vi "Measurement Logic.vi"() -> ()   [LabVIEW 2021, in "Load Transient Response with Pin Map.lvlib"]
uses:
  Load Transient Response with Pin Map.lvlib
  <vilib>/Plug-In SDKs/Measurements/Measure Call Context/Measure Call Context.lvclass
  Measurement Configuration.ctl
  <instrlib>/niScope/Controls/niScope vertical coupling.ctl
  Measurement Results.ctl
  subVIs/Reference values.ctl
  <vilib>/Plug-In SDKs/Clients/Session Management V1/Session Reservation/Session Reservation.lvclass
  common/Instrument Control/Scope/TClk/Instrument Info.ctl
  common/Instrument Control/Scope Parameters.ctl
  <instrlib>/niDCPower/nidcpower.llb/niDCPower Sense.ctl
  <instrlib>/niDCPower/nidcpower.llb/niDCPower Source Mode.ctl
  <instrlib>/niDCPower/nidcpower.llb/niDCPower Wait For Event - Event.ctl
  <instrlib>/niDCPower/nidcpower.llb/niDCPower Output Function.ctl
  <instrlib>/niDCPower/nidcpower.llb/niDCPower Aperture Time Units.ctl
  <vilib>/Plug-In SDKs/Measurements/Measure Call Context/Reserve Sessions - NPin.vi
  <vilib>/Plug-In SDKs/Sessions/niDCPower/Initialize Sessions - NSess.vi
  <vilib>/Plug-In SDKs/Sessions/niDCPower/Get Connections - 1Pin 1Conn.vi
  <vilib>/Plug-In SDKs/Sessions/niScope/Initialize Sessions - NSess.vi
  <vilib>/Plug-In SDKs/Sessions/niScope/Get Connections - NPin MConn.vi
  <instrlib>/niScope/Configure/Trigger/niScope Configure Trigger Digital.vi
  <instrlib>/niDCPower/nidcpower.llb/niDCPower Configure Digital Edge Measure Trigger With Channels.vi
  <vilib>/Plug-In SDKs/Sessions/niDCPower/NI Session Management niDCPower.lvlib
  <vilib>/Plug-In SDKs/Sessions/niScope/NI Session Management niScope.lvlib
  common/PMIC Common.lvlib
panel:
  out "measurement results":T1={"Status"="Empty", "dt"=0.0, "Load voltages"=[0.0], "Load currents"=[0.0], "Undershoot load voltage"=0.0, "Overshoot load voltage"=0.0, "waveform pins"=[], "waveform sites"=[], "waveform t0 array"=[], "waveform dt array"=[], "waveform length array"=[], "concatenated waveform Y"=[]}
  in  "measurement configuration":T2={"Mode of operation"=enum."Perform measurement", "DUT setup time"=1.2, "Nominal output voltage"=32.0, "Source pin name"="Lorem ipsum dolor sit", "Source sense"=64, "Source current limit"=64.0, "Source voltage level"=-32.0, "Source transient response"=-32, "Source voltage gain bandwidth"=-64.0, "Source voltage compensation frequency"=-64.0, "Source voltage pole-zero ratio"=1.0, "Load pin name"="Lorem ipsum dolor sit", "Load sense"=1, "Load voltage limit range"=1.0, "Load current level range"=40.0, "Load sample rate"=1800000.0, "Load current set point 1"=4.0, "Load current set point 2"=14.0, "Load current delay t1"=0.001, "Load current pulse duration"=0.001, "Load current delay t2"=0.001, "Load current rising slew rate"=24.0, "Load current falling slew rate"=24.0, "Load transient response"=1042, "Load current gain bandwidth"=14000.0, "Load current compensation frequency"=180000.0, "Load current pole-zero ratio"=0.3, "Pin Names for Scope"=[], "vertical range"=[], "vertical offset"=[], "probe attenuation"=[], "vertical coupling"=[], "input impedance"=[], "max input frequency"=[], "min record length"=[], "channel enabled"=[], "enforce realtime"=[], "reference position"=[], "min sample rate"=[]} {"input impedance" items=["1 mega ohm"=0, "50 ohms"=2]; "vertical coupling" items=["AC", "DC", "Ground"]; "Load transient response" items=["Slow"=1041, "Normal"=1038, "Fast"=1039, "Custom"=1042]; "Load current falling slew rate" format="%#_6p"; "Load current rising slew rate" format="%#_6p"; "Load current level range" format="%#_6p"; "Load voltage limit range" format="%#_6p"; "Load sense" items=["Red", "Green", "Blue"]; "Source transient response" items=["Slow"=1041, "Normal"=1038, "Fast"=1039, "Custom"=1042]; "Source sense" items=["Local"=1008, "Remote"=1009]; "Nominal output voltage" format="%#_6pV"}
  out "measure call context out":refnum<class "Measure Call Context.lvclass">
  in  "measure call context in":refnum<class "Measure Call Context.lvclass">
  out "error out":errorcluster
  in  "error in":errorcluster
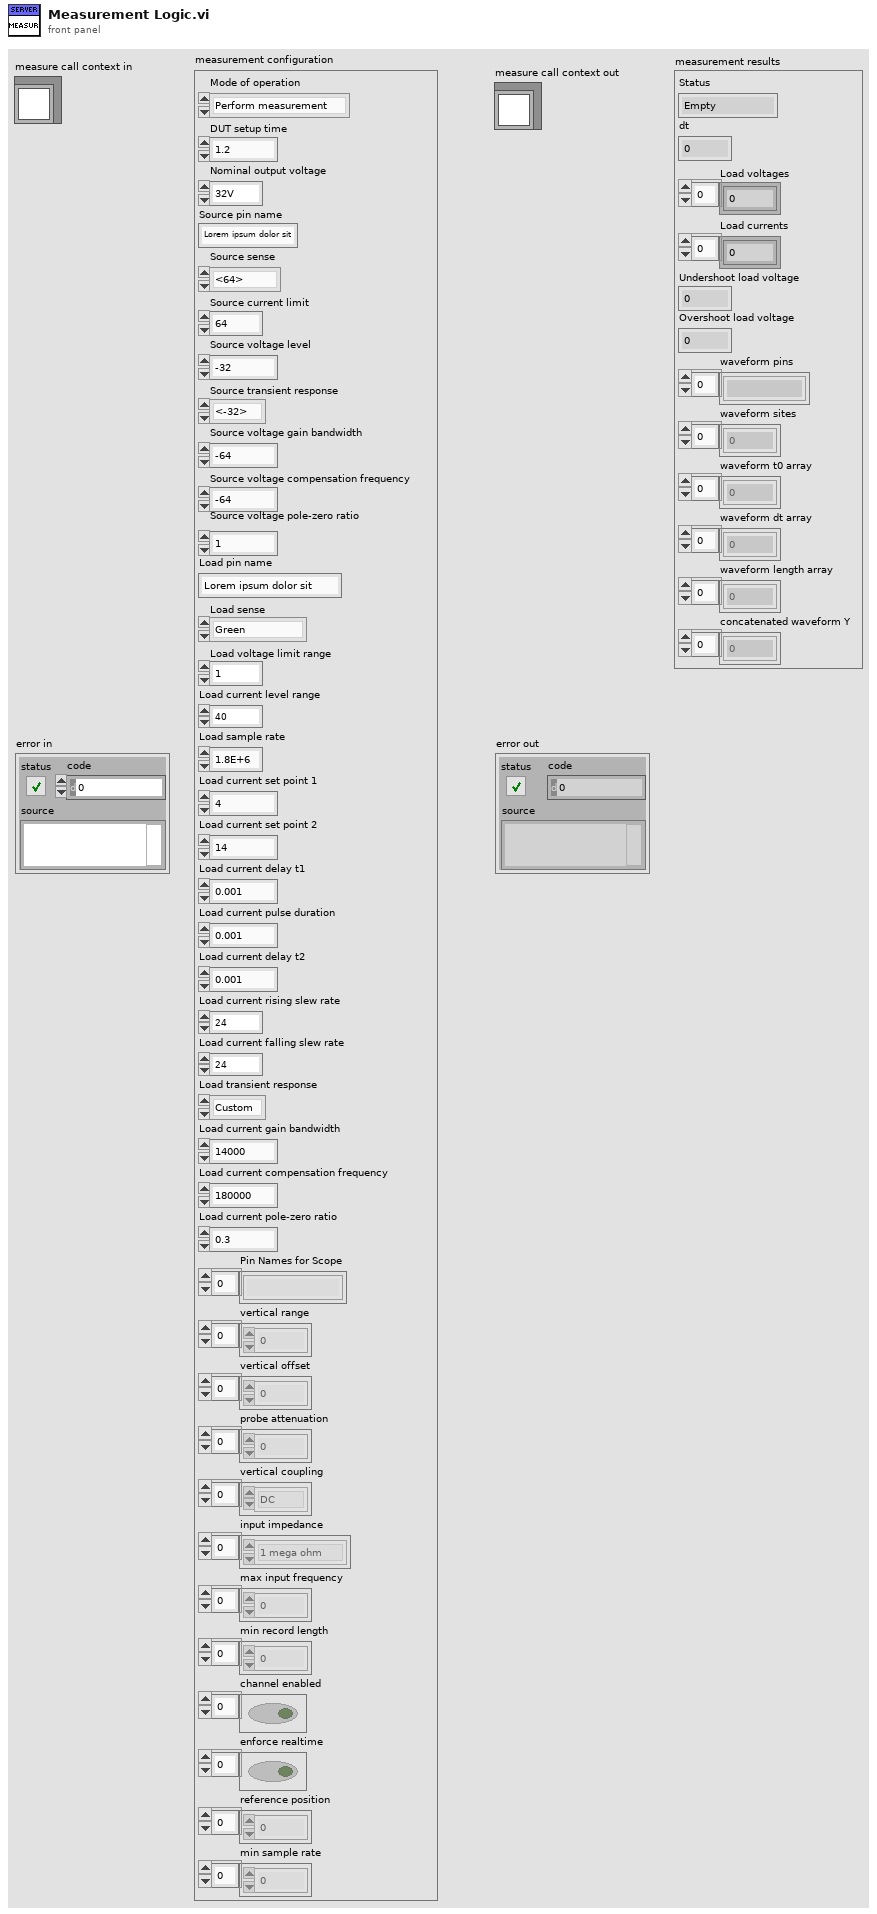
[diagram p1: front panel]
types:
  T1 = typedef "Load Transient Response with Pin Map.lvlib/Measurement Results.ctl" = cluster{"Status":string, "dt":dbl, "Load voltages":dbl[], "Load currents":dbl[], "Undershoot load voltage":dbl, "Overshoot load voltage":dbl, "waveform pins":string[], "waveform sites":i32[], "waveform t0 array":dbl[], "waveform dt array":dbl[], "waveform length array":i32[], "concatenated waveform Y":dbl[]}
  T2 = typedef "Load Transient Response with Pin Map.lvlib/Measurement Configuration.ctl" = cluster{"Mode of operation":enum32{"Power on the DUT", "Perform measurement", "Power off the DUT"}, "DUT setup time":dbl, "Nominal output voltage":dbl, "Source pin name":string, "Source sense":i32, "Source current limit":dbl, "Source voltage level":dbl, "Source transient response":i32, "Source voltage gain bandwidth":dbl, "Source voltage compensation frequency":dbl, "Source voltage pole-zero ratio":dbl, "Load pin name":string, "Load sense":i32, "Load voltage limit range":dbl, "Load current level range":dbl, "Load sample rate":dbl, "Load current set point 1":dbl, "Load current set point 2":dbl, "Load current delay t1":dbl, "Load current pulse duration":dbl, "Load current delay t2":dbl, "Load current rising slew rate":dbl, "Load current falling slew rate":dbl, "Load transient response":i32, "Load current gain bandwidth":dbl, "Load current compensation frequency":dbl, "Load current pole-zero ratio":dbl, "Pin Names for Scope":string[], "vertical range":dbl[], "vertical offset":dbl[], "probe attenuation":dbl[], "vertical coupling":T3[], "input impedance":u32[], "max input frequency":dbl[], "min record length":i32[], "channel enabled":bool[], "enforce realtime":bool[], "reference position":dbl[], "min sample rate":dbl[]}
  T3 = typedef "niScope vertical coupling.ctl" = i32
  T4 = typedef "Load Transient Response with Pin Map.lvlib/Reference values.ctl" = cluster{"dcpower session reservation":refnum<class "Session Reservation.lvclass">, "Source out":refnum<k15>, "Source channel name":string, "Load out":refnum<k15>, "Load channel name":string, "No of samples to fetch":i32, "Source voltage level":dbl, "Source current limit":dbl, "Measure terminal name":string, "Scope ref trigger source":string, "scope session reservation":refnum<class "Session Reservation.lvclass">, "Scope handles":refnum<k15>[][], "connection map":map{string, T5[]}, "instrument info map array":map{string, cluster{"channel":string, "siteNumber":i32, "pin":string, "Scope Parameters":T6}[]}[], "Enable TClk":bool, "Number of records":i32, "Measurement Results":T1}
  T5 = typedef "PMIC Common.lvlib/Instrument Info.ctl" = cluster{"instrument":string, "channel":string, "siteNumber":i32}
  T6 = typedef "PMIC Common.lvlib/Scope Parameters.ctl" = cluster{"vertical range":dbl, "vertical offset":dbl, "probe attenuation":dbl, "vertical coupling":T3, "channel enabled":bool, "input impedance":u32, "maximum input frequency":dbl, "min sample rate":dbl, "reference position":dbl, "min record length":i32, "number of records":i32, "enforce realtime":bool}
  T7 = enum32{"Power on the DUT", "Perform measurement", "Power off the DUT"}
  T8 = typedef "niDCPower Wait For Event - Event.ctl" = i32
  T9 = typedef "niDCPower Source Mode.ctl" = i32
  T10 = typedef "niDCPower Sense.ctl" = i32
  T11 = typedef "NI Session Management niDCPower.lvlib/Connection with Session.ctl" = cluster{"connection":T12, "session":refnum<k15>}
  T12 = typedef "NI Session Management V1 Client.lvlib/Session Reservation.lvclass/Connection.ctl" = cluster{"pin or relay name":string, "site":i32, "instrument type id":string, "channel":string}
  T13 = typedef "niDCPower Output Function.ctl" = i32
  T14 = cluster{"Numeric":dbl, "Numeric":dbl, "Numeric":dbl, "vertical coupling":T3, "Boolean":bool, "input impedance":u32, "Numeric":dbl, "Numeric":dbl, "Numeric":dbl, "Numeric":i32, "Number of records":i32, "Boolean":bool}[]
  T15 = typedef "NI Session Management niScope.lvlib/Connection with Session.ctl" = cluster{"connection":T12, "session":refnum<k15>}
  T16 = typedef "NI Measurement Plug-In SDK.lvlib/Pin Map Context.ctl" = cluster{"pin map id":string, "sites":i32[]}
  T17 = map{string, cluster{"channel":string, "siteNumber":i32, "pin":string, "Scope Parameters":T6}[]}[]
  T18 = typedef "niDCPower Aperture Time Units.ctl" = i32
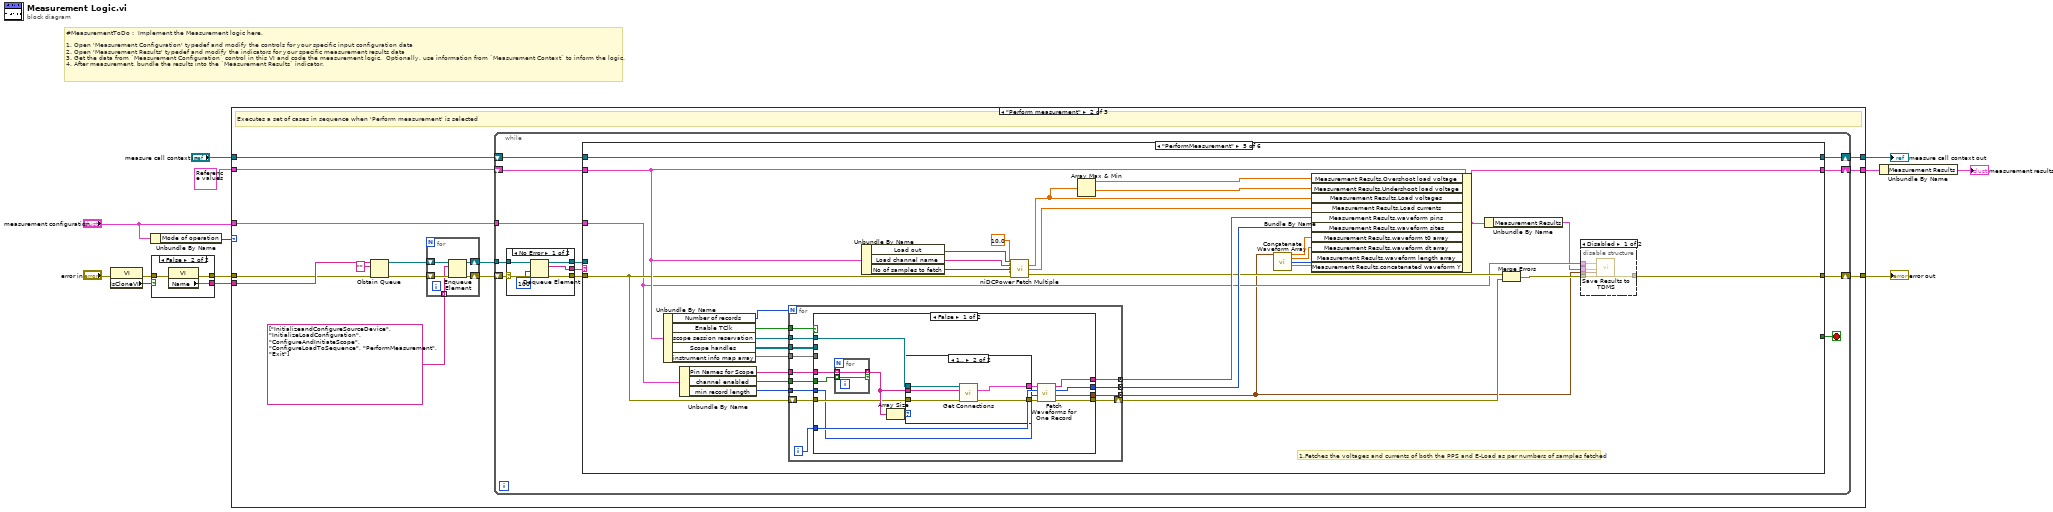
[diagram p0: block diagram]
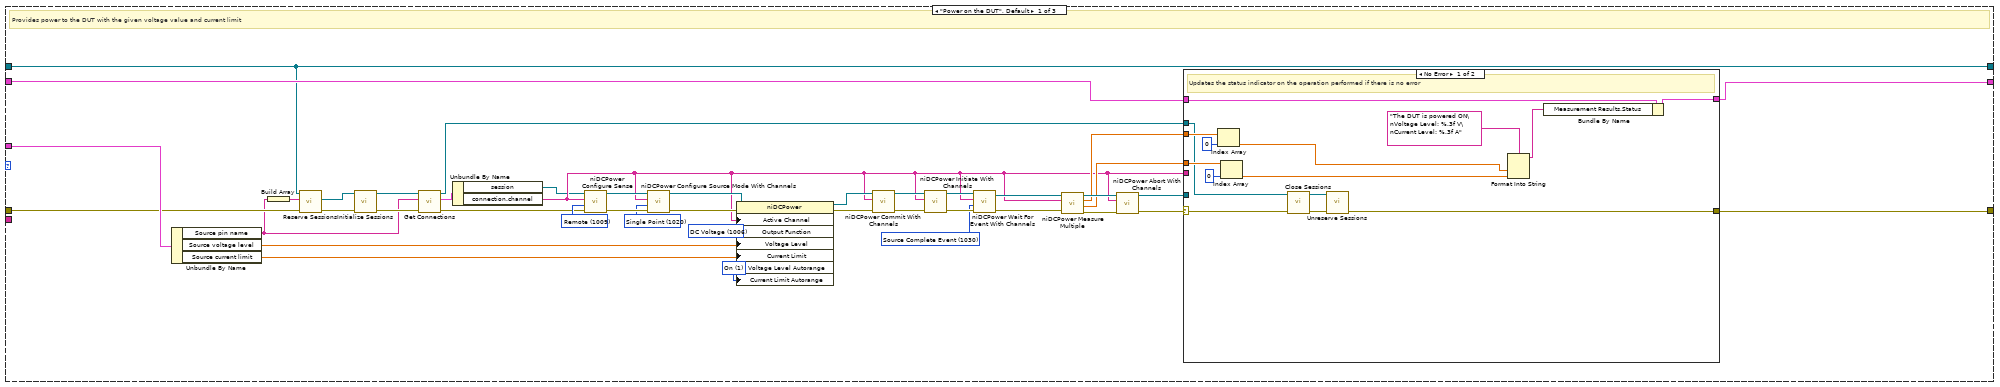
[diagram p2: hidden frame]
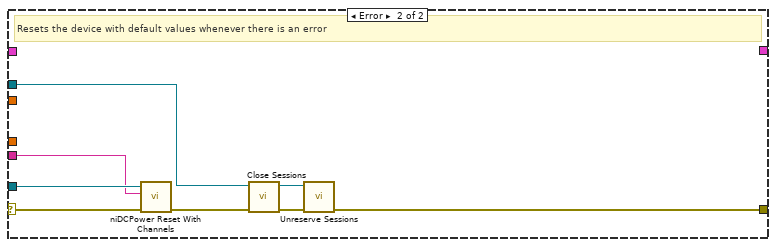
[diagram p3: hidden frame]
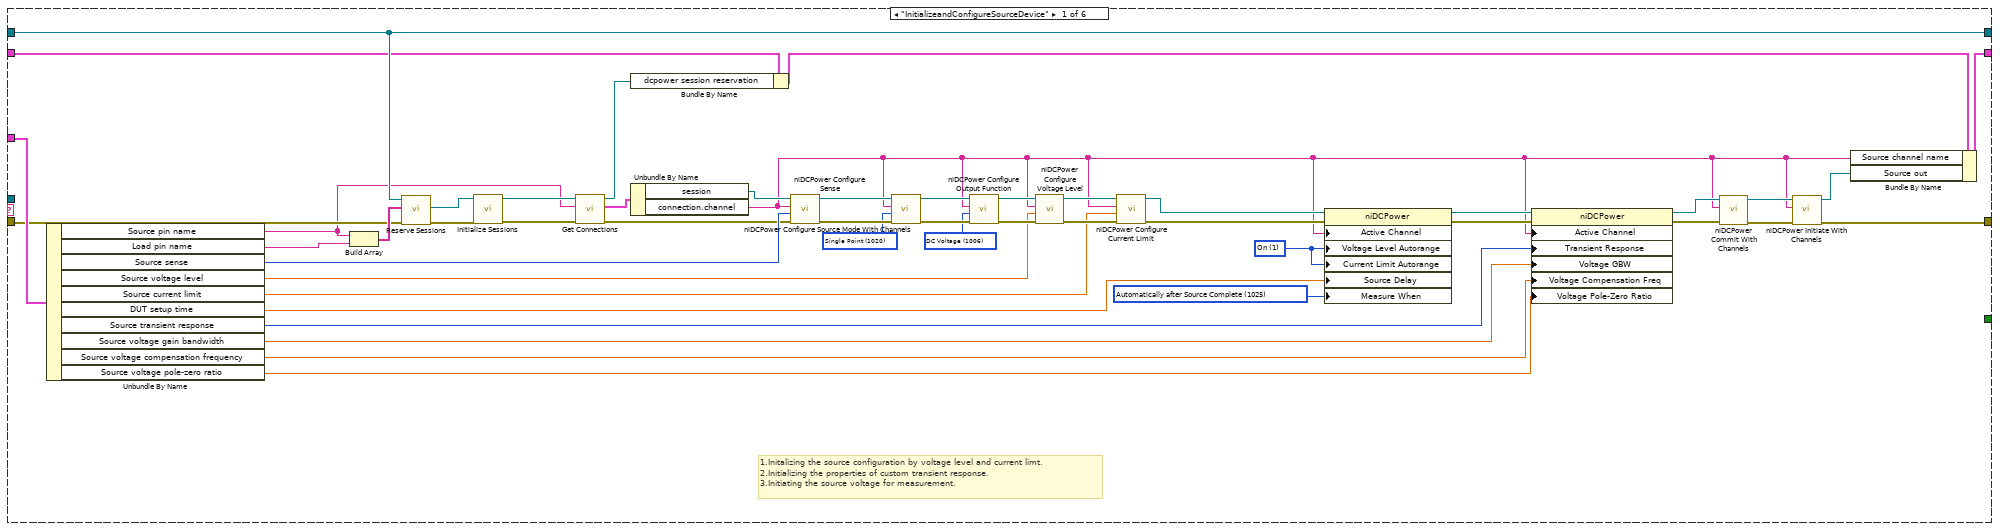
[diagram p4: hidden frame]
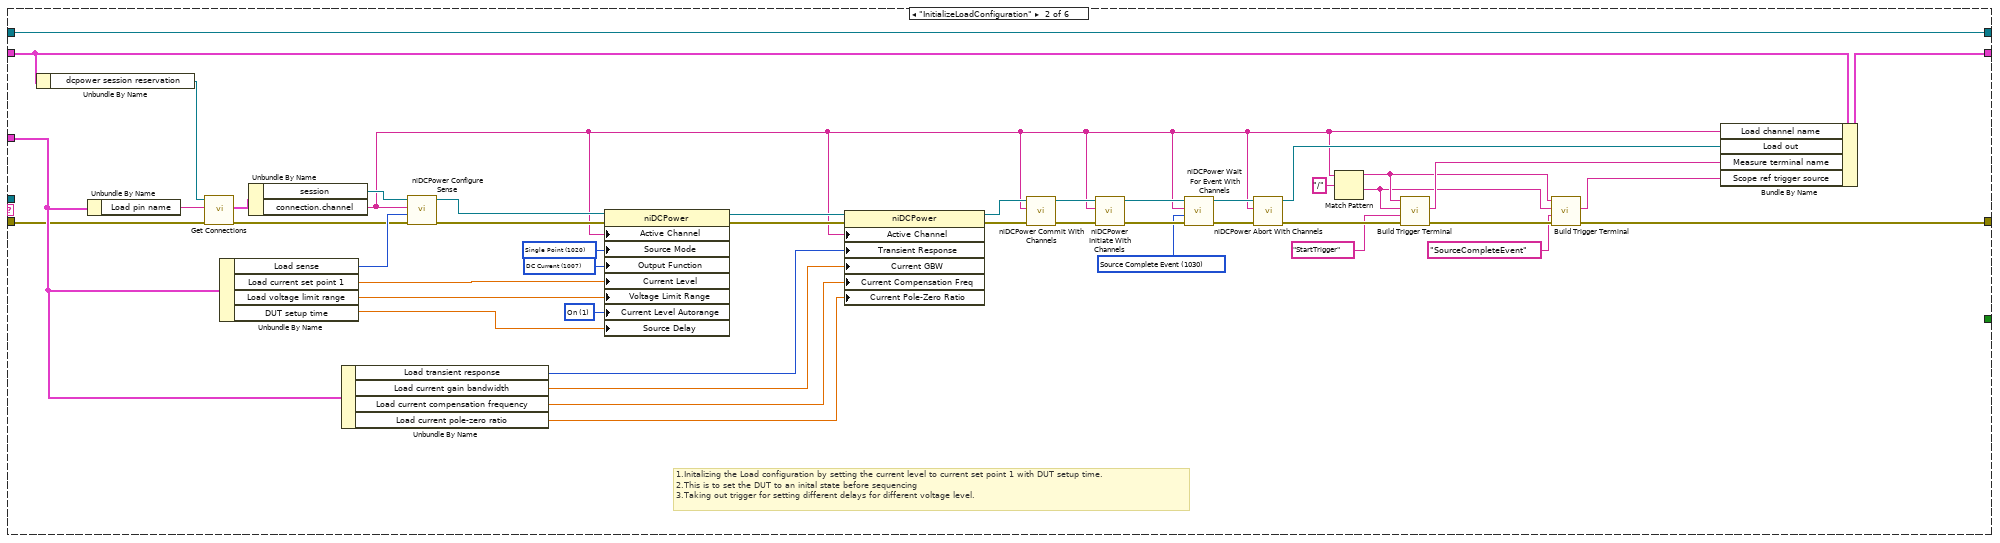
[diagram p5: hidden frame]
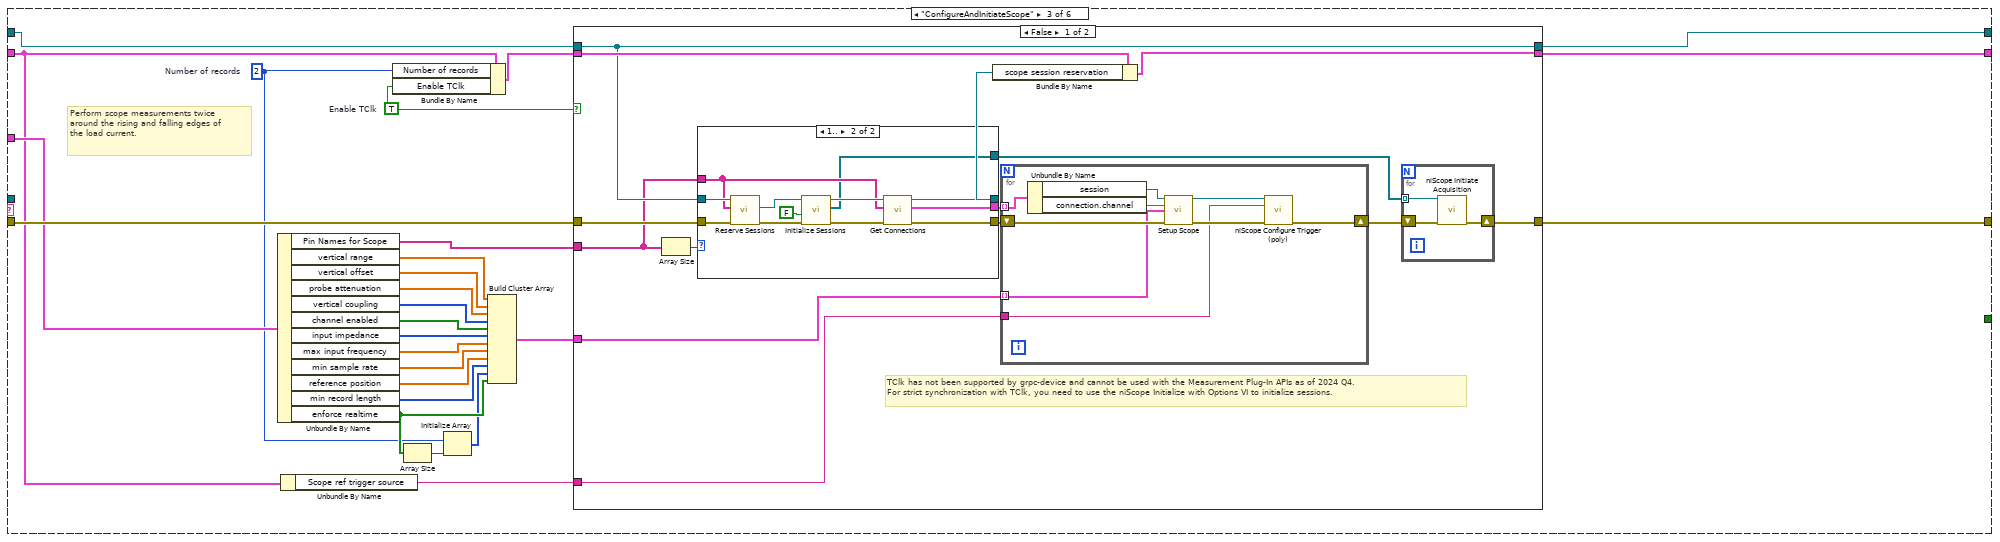
[diagram p6: hidden frame]
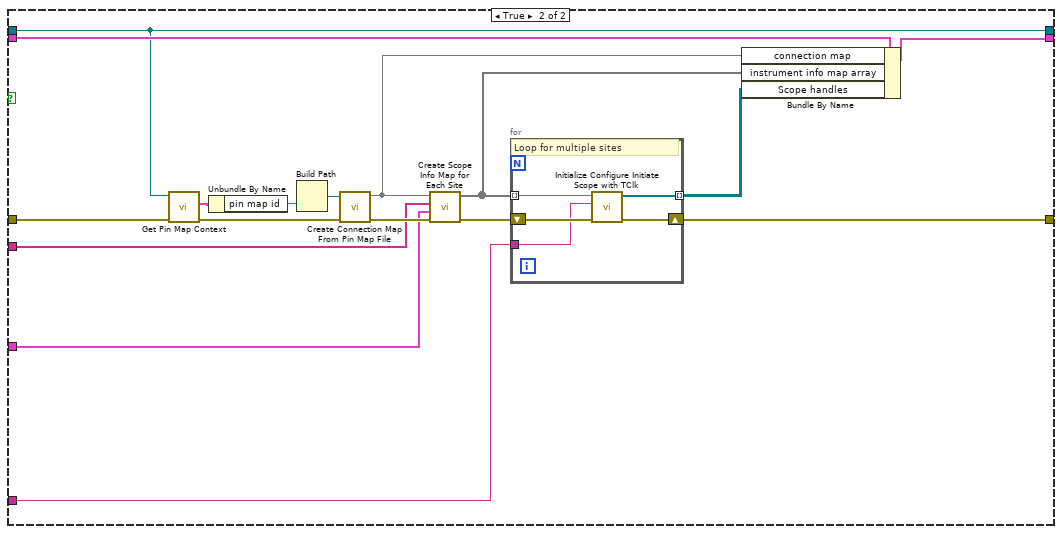
[diagram p8: hidden frame]
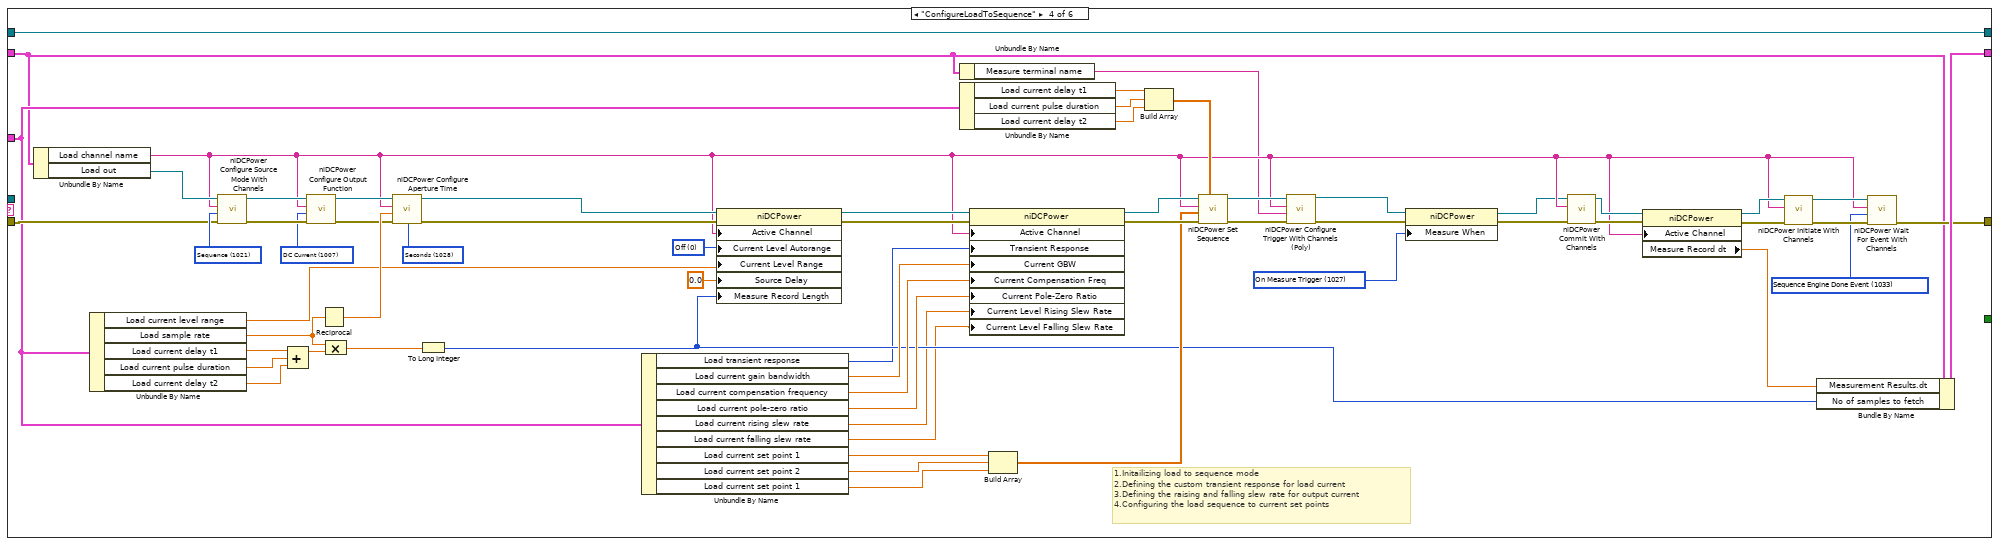
[diagram p9: hidden frame]
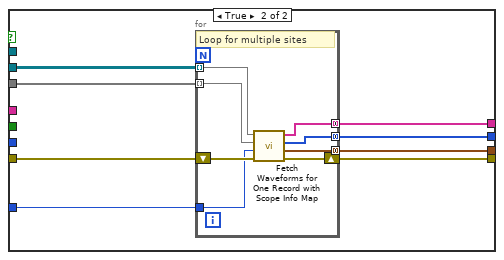
[diagram p12: hidden frame]
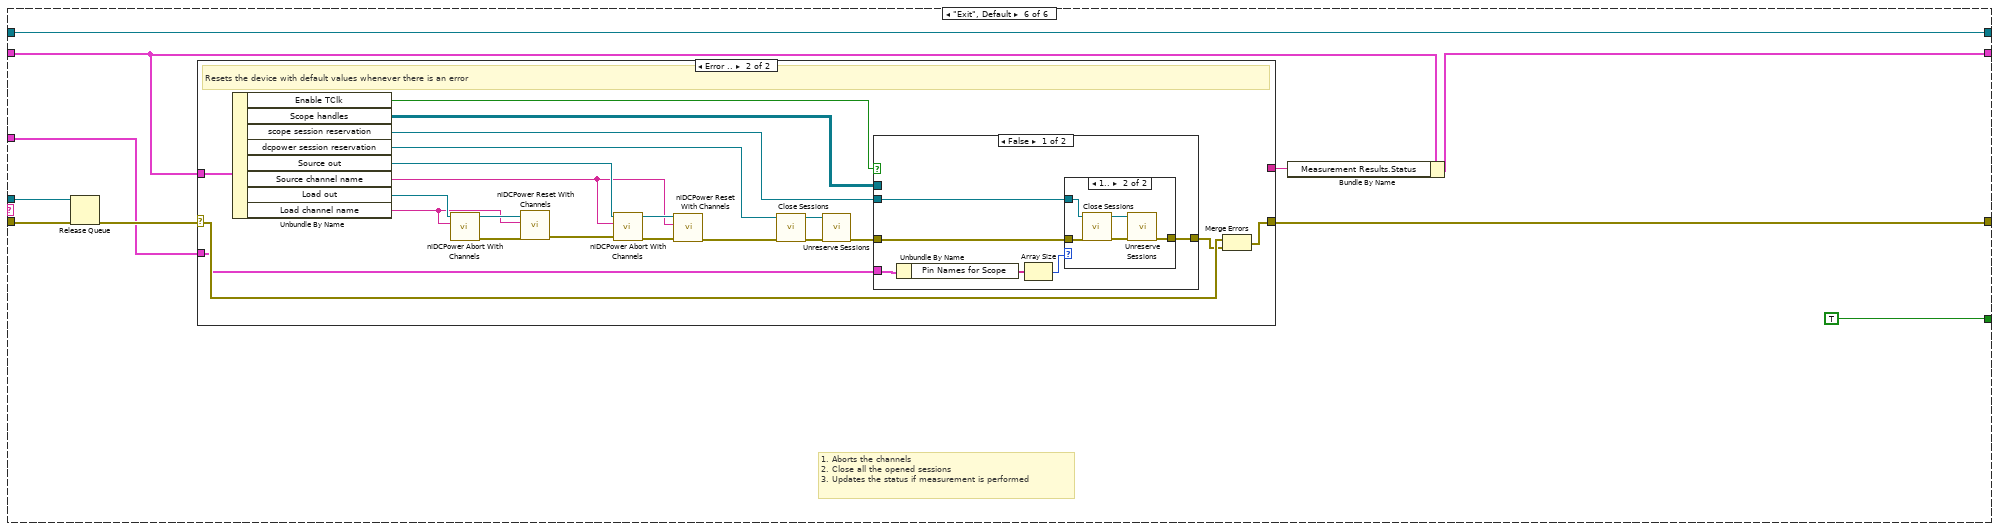
[diagram p13: hidden frame]
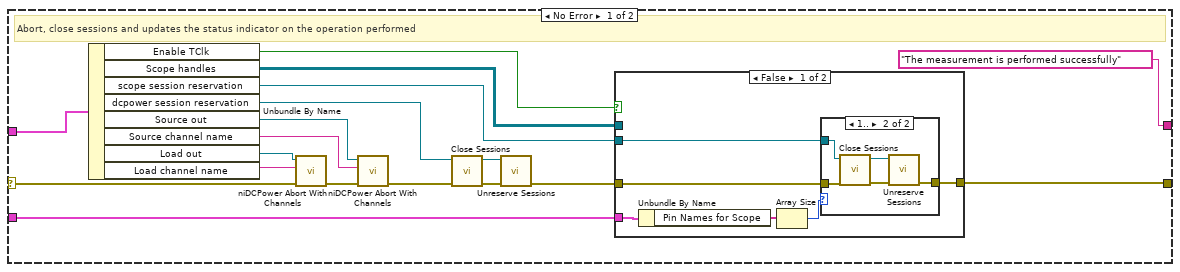
[diagram p14: hidden frame]
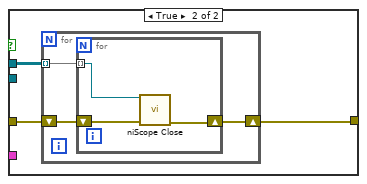
[diagram p16: hidden frame]
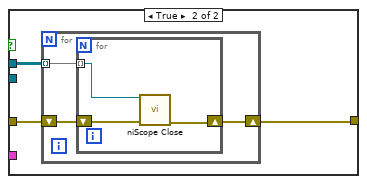
[diagram p18: hidden frame]
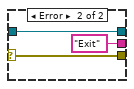
[diagram p19: hidden frame]
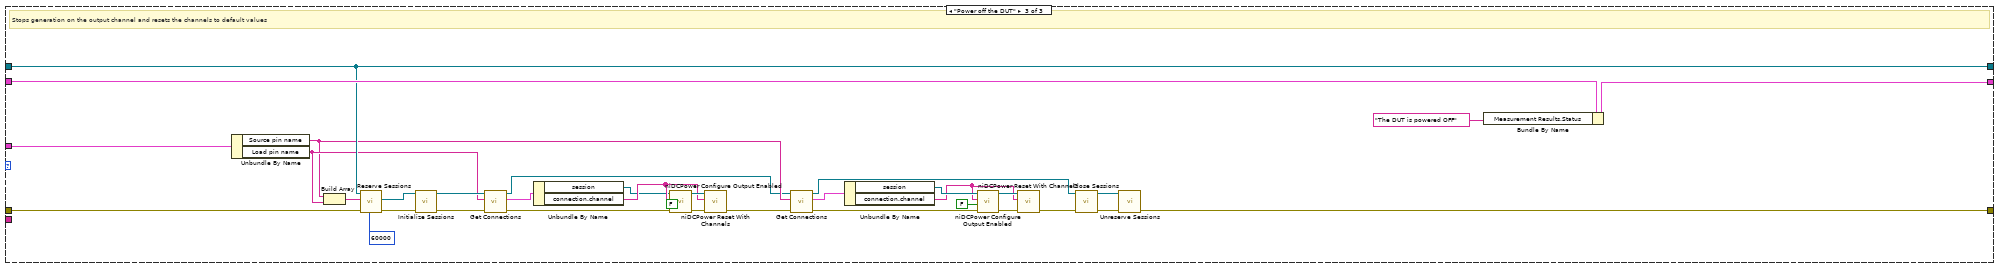
[diagram p20: hidden frame]
diagram:
  # "#MeasurementToDo :  Implement the Measurement logic here.\n\n1. Open 'Measurement Configuration' typedef and modify the controls for your specific input configuration data\n2. Open 'Measurement Results' typedef and modify the indicators for your specific measurement results data\n3. Get the data from `Measurement Configuration` control in this VI and code the measurement logic.  Optionally, use information from `Measurement Context` to inform the logic.\n4. After measurement, bundle the results into the `Measurement Results` indicator."
  n1 = property class="VI"(error in="error in") -> (error out=w12:errorcluster, "IsCloneVI"=w13:bool)  [unwired: 1 in, 1 out]
  n2 = Unbundle By Name("measurement configuration") -> ("Mode of operation"=w8:T7)
  n3 = case shown="False" w13 {
    tunnel: [w16 w19] -> w9
    tunnel: [w15 w18] -> w7
    tunnel: w12 -> [w14 w17]
    frame True {
      n4 = property class="VI"(error in=w14) -> (error out=w16:errorcluster, "Clone Name"=w15:string)  [unwired: 1 in, 1 out]
    }
    frame False {
      n5 = property class="VI"(error in=w17) -> (error out=w19:errorcluster, "Name"=w18:string)  [unwired: 1 in, 1 out]
    }
  }
  n6 = case shown="\"Perform measurement\"" w8 {
    tunnel: T4 {"dcpower session reservation"=refnum, "Source out"="", "Source channel name"="", "Load out"="", "Load channel name"="", "No of samples to fetch"=1, "Source voltage level"=0.0, "Source current limit"=0.0, "Measure terminal name"="", "Scope ref trigger source"="", "scope session reservation"=refnum, "Scope handles"=[], "connection map"={}, "instrument info map array"=[], "Enable TClk"=FALSE, "Number of records"=2, "Measurement Results"={"Status"="Empty", "dt"=0.0, "Load voltages"=[], "Load currents"=[], "Undershoot load voltage"=0.0, "Overshoot load voltage"=0.0, "waveform pins"=[], "waveform sites"=[], "waveform t0 array"=[], "waveform dt array"=[], "waveform length array"=[], "concatenated waveform Y"=[]}} -> [w41 w98 w580]
    tunnel: "measure call context in" -> [w28 w97 w570]
    tunnel: [w34 w96 w558] -> w1
    tunnel: [w28 w95 w570] -> w2
    tunnel: [w33 w94 w578] -> w10
    tunnel: "measurement configuration" -> [w44 w93 w581]
    tunnel: w9 -> [w26 w86 w572]
    tunnel: w7 -> [_ w89 _]
    frame "Power on the DUT", Default {
      w47 = 1 items=["Off", "On"] ("Source:DC Voltage:Voltage Level Autorange")
      w46 = T8 1030 items=["Source Complete Event"=1030, "Measure Complete Event"=1031, "Sequence Iteration Complete Event"=1032, "Sequence Engine Done Event"=1033, "Pulse Complete Event"=1051, "Ready For Pulse Trigger Event"=1052] ("event")
      w45 = T9 1020 items=["Single Point"=1020, "Sequence"=1021] ("source mode")
      w48 = 1006 items=["DC Voltage"=1006, "DC Current"=1007, "Pulse Voltage"=1049, "Pulse Current"=1050] ("Source:Output Function")
      w49 = T10 1009 items=["Local"=1008, "Remote"=1009] ("sense")
      # "Provides power to the DUT with the given voltage value and current limit"
      n7 = Unbundle By Name(w44) -> ("Source pin name"=w24:string, "Source voltage level"=w60:dbl, "Source current limit"=w61:dbl)
      n8 = Build Array(w24) -> (w27:string[])
      n9 = call-poly <vilib>:"Reserve Sessions.vi"("error in"=w26, "pin or relay names"=w27, "measurement context in"=w28) -> ("error out"=w32:errorcluster, "session reservation out"=w31:refnum<class "Session Reservation.lvclass">)  [unwired: 6 in, 1 out]
      n10 = call-poly <vilib>:"Initialize Sessions.vi"("error in"=w32, "session reservation in"=w31) -> ("error out"=w30:errorcluster, "session reservation out"=w29:refnum<class "Session Reservation.lvclass">)  [unwired: 6 in, 2 out]
      n11 = call-poly <vilib>:"Get Connections.vi"("error in"=w30, "pin or relay name"=w24, "session reservation in"=w29) -> ("error out"=w23:errorcluster, "connection"=w25:T11, "session reservation out"=w20:refnum<class "Session Reservation.lvclass">)  [unwired: 6 in]
      n12 = Unbundle By Name(w25) -> ("session"=w21:refnum<k15>, "connection.channel"=w22:string)
      n13 = call <instrlib>:"niDCPower Configure Sense.vi"("error in (no error)"=w23, "sense"=w49, "channel name"=w22, "instrument handle"=w21) -> ("error out"=w55:errorcluster, "instrument handle out"=w57:refnum<k15>)  [unwired: 6 in]
      n14 = call <instrlib>:"niDCPower Configure Source Mode With Channels.vi"("error in (no error)"=w55, "source mode"=w45, "channel name"=w22, "instrument handle"=w57) -> ("error out"=w54:errorcluster, "instrument handle out"=w56:refnum<k15>)  [unwired: 6 in]
      n15 = property class="niDCPower"(reference=w56, error in=w54, "Active Channel"=w22, "Output Function"=w48, "Voltage Level"=w60, "Current Limit"=w61, "Voltage Level Autorange"=w47, "Current Limit Autorange"=w47) -> (reference out=w53:refnum<k15>, error out=w52:errorcluster)
      n16 = call <instrlib>:"niDCPower Commit With Channels.vi"("error in (no error)"=w52, "channel name"=w22, "instrument handle"=w53) -> ("error out"=w50:errorcluster, "instrument handle out"=w51:refnum<k15>)  [unwired: 7 in]
      n17 = call <instrlib>:"niDCPower Initiate With Channels.vi"("error in (no error)"=w50, "channel name"=w22, "instrument handle"=w51) -> ("error out"=w59:errorcluster, "instrument handle out"=w58:refnum<k15>)  [unwired: 7 in]
      n18 = call <instrlib>:"niDCPower Wait For Event With Channels.vi"("error in (no error)"=w59, "event"=w46, "channel name"=w22, "instrument handle"=w58) -> ("error out"=w38:errorcluster, "instrument handle out"=w40:refnum<k15>)  [unwired: 6 in]
      n19 = call <instrlib>:"niDCPower Measure Multiple.vi"("error in (no error)"=w38, "channel name"=w22, "instrument handle"=w40) -> ("error out"=w37:errorcluster, "current measurements"=w35:dbl[], "voltage measurements"=w36:dbl[], "instrument handle out"=w39:refnum<k15>)  [unwired: 5 in]
      n20 = call <instrlib>:"niDCPower Abort With Channels.vi"("error in (no error)"=w37, "channel name"=w22, "instrument handle"=w39) -> ("error out"=w43:errorcluster, "instrument handle out"=w42:refnum<k15>)  [unwired: 7 in]
      n21 = case shown="No Error" w43 {
        selector: w43 -> [w63 w83]
        tunnel: [w64 w79] -> w34
        tunnel: w42 -> [_ w84]
        tunnel: w22 -> [_ w82]
        tunnel: w41 -> [w76 _]
        tunnel: [w75 _] -> w33
        tunnel: w36 -> [w72 _]
        tunnel: w35 -> [w71 _]
        tunnel: w20 -> [w62 w77]
        frame No Error {
          # "Updates the status indicator on the operation performed if there is no error"
          n22 = Index Array(array=w72, index=0) -> (element=w68:dbl)
          n23 = Index Array(array=w71, index=0) -> (element=w67:dbl)
          n24 = call <vilib>:"Close Sessions.vi"("error in"=w63, "session reservation in"=w62) -> ("error out"=w65:errorcluster, "session reservation out"=w66:refnum<class "Session Reservation.lvclass">)  [unwired: 8 in]
          n25 = call <vilib>:"Unreserve Sessions.vi"("error in"=w65, "session reservation in"=w66) -> ("error out"=w64:errorcluster)  [unwired: 9 in]
          n26 = Format Into String(format string="The DUT is powered ON\nVoltage Level: %.3f V\nCurrent Level: %.3f A" ("message"), w68, w67) -> (resulting string=w73:string)  [unwired: 2 in, 1 out]
          n27 = Bundle By Name(cluster=w76, "Measurement Results.Status"=w73) -> (w75:T4)
        }
        frame Error {
          # "Resets the device with default values whenever there is an error"
          n28 = call <instrlib>:"niDCPower Reset With Channels.vi"("error in (no error)"=w83, "channel name"=w82, "instrument handle"=w84) -> ("error out"=w78:errorcluster)  [unwired: 7 in, 1 out]
          n29 = call <vilib>:"Close Sessions.vi"("error in"=w78, "session reservation in"=w77) -> ("error out"=w80:errorcluster, "session reservation out"=w81:refnum<class "Session Reservation.lvclass">)  [unwired: 8 in]
          n30 = call <vilib>:"Unreserve Sessions.vi"("error in"=w80, "session reservation in"=w81) -> ("error out"=w79:errorcluster)  [unwired: 9 in]
        }
      }
    }
    frame "Perform measurement" {
      # "Executes a set of cases in sequence when 'Perform measurement' is selected"
      n31 = Obtain Queue(name (unnamed)=w89, element data type="", error in (no error)=w86) -> (queue out=w88:refnum<queue>, error out=w87:errorcluster)  [unwired: 2 in, 1 out]
      n32 = for {
        tunnel: string[] ["InitializeandConfigureSourceDevice", "InitializeLoadConfiguration", "ConfigureAndInitiateScope", "ConfigureLoadToSequence", "PerformMeasurement", "Exit"] ("Step sequence") -> [w99] mode=indexing
        shift-right: [w102] -> w90
        shift-left: w88 -> [w101]
        shift-right: [w103] -> w91
        shift-left: w87 -> [w100]
        n33 = Enqueue Element(queue=w101, element=w99, error in (no error)=w100) -> (queue out=w102:refnum<queue>, error out=w103:errorcluster)  [unwired: 1 in, 1 out]
      }
      n34 = while {
        tunnel: w90 -> [w115]
        shift-right: [w108] -> w96
        shift-left: w91 -> [w114]
        tunnel: w93 -> [w110]
        shift-right: [w105] -> w95
        shift-left: w97 -> [w106]
        shift-right: [w104] -> w94
        shift-left: w98 -> [w107]
        stop <- w109 stop-if-true
        n35 = case shown="No Error" w114 {
          selector: w114 -> [w544 w548]
          tunnel: w115 -> [w546 w547]
          tunnel: [w545 "Exit" ("t")] -> w113
          tunnel: [w543 w548] -> w111
          tunnel: [w541 w547] -> w112
          frame No Error {
            n36 = Dequeue Element(queue=w546, timeout in ms (-1)=100, error in (no error)=w544) -> (queue out=w541:refnum<queue>, element=w545:string, error out=w543:errorcluster)  [unwired: 1 out]
          }
          frame Error {
          }
        }
        n37 = case shown="\"PerformMeasurement\"" w113 {
          tunnel: w112 -> [_ _ _ _ _ w456]
          tunnel: w111 -> [w123 w176 w235 w330 w377 w455]
          tunnel: w110 -> [w149 w195 w216 w311 w364 w449]
          tunnel: [_ _ _ _ _ TRUE] -> w109
          tunnel: [w134 w168 w234 w323 w365 w451] -> w108
          tunnel: w107 -> [w118 w178 w211 w303 w382 w450]
          tunnel: w106 -> [w125 w188 w232 w324 w391 w457]
          tunnel: [w125 w188 w231 w324 w391 w457] -> w105
          tunnel: [w141 w189 w233 w329 w362 w453] -> w104
          frame "InitializeandConfigureSourceDevice" {
            w144 = 1025 items=["Automatically after Source Complete"=1025, "On Demand"=1026, "On Measure Trigger"=1027] ("Measurement:Advanced:Measure When")
            w150 = 1 items=["Off", "On"] ("Source:DC Voltage:Current Limit Autorange")
            w151 = T13 1006 items=["DC Voltage"=1006, "DC Current"=1007, "Pulse Voltage"=1049, "Pulse Current"=1050] ("output function")
            w152 = T9 1020 items=["Single Point"=1020, "Sequence"=1021] ("source mode")
            # "1.Initalizing the source configuration by voltage level and current limt.\n2.Initializing the properties of custom transient response.\n3.Initiating the source voltage for measurement."
            n38 = Unbundle By Name(w149) -> ("Source pin name"=w119:string, "Load pin name"=w120:string, "Source sense"=w133:i32, "Source voltage level"=w136:dbl, "Source current limit"=w137:dbl, "DUT setup time"=w138:dbl, "Source transient response"=w135:i32, "Source voltage gain bandwidth"=w143:dbl, "Source voltage compensation frequency"=w140:dbl, "Source voltage pole-zero ratio"=w132:dbl)
            n39 = Build Array(w119, w120) -> (w126:string[])
            n40 = call-poly <vilib>:"Reserve Sessions.vi"("error in"=w123, "pin or relay names"=w126, "measurement context in"=w125) -> ("error out"=w131:errorcluster, "session reservation out"=w130:refnum<class "Session Reservation.lvclass">)  [unwired: 6 in, 1 out]
            n41 = call-poly <vilib>:"Initialize Sessions.vi"("error in"=w131, "session reservation in"=w130) -> ("error out"=w129:errorcluster, "session reservation out"=w128:refnum<class "Session Reservation.lvclass">)  [unwired: 6 in, 2 out]
            n42 = call-poly <vilib>:"Get Connections.vi"("error in"=w129, "pin or relay name"=w119, "session reservation in"=w128) -> ("error out"=w124:errorcluster, "connection"=w127:T11, "session reservation out"=w117:refnum<class "Session Reservation.lvclass">)  [unwired: 6 in]
            n43 = Bundle By Name(cluster=w118, "dcpower session reservation"=w117) -> (w116:T4)
            n44 = Unbundle By Name(w127) -> ("session"=w122:refnum<k15>, "connection.channel"=w121:string)
            n45 = call <instrlib>:"niDCPower Configure Sense.vi"("error in (no error)"=w124, "sense"=w133, "channel name"=w121, "instrument handle"=w122) -> ("error out"=w162:errorcluster, "instrument handle out"=w163:refnum<k15>)  [unwired: 6 in]
            n46 = call <instrlib>:"niDCPower Configure Source Mode With Channels.vi"("error in (no error)"=w162, "source mode"=w152, "channel name"=w121, "instrument handle"=w163) -> ("error out"=w153:errorcluster, "instrument handle out"=w154:refnum<k15>)  [unwired: 6 in]
            n47 = call <instrlib>:"niDCPower Configure Output Function.vi"("error in (no error)"=w153, "output function"=w151, "channel name"=w121, "instrument handle"=w154) -> ("error out"=w156:errorcluster, "instrument handle out"=w157:refnum<k15>)  [unwired: 6 in]
            n48 = call <instrlib>:"niDCPower Configure Voltage Level.vi"("error in (no error)"=w156, "voltage level"=w136, "channel name"=w121, "instrument handle"=w157) -> ("error out"=w159:errorcluster, "instrument handle out"=w158:refnum<k15>)  [unwired: 6 in]
            n49 = call <instrlib>:"niDCPower Configure Current Limit.vi"("error in (no error)"=w159, "current limit"=w137, "channel name"=w121, "instrument handle"=w158) -> ("error out"=w155:errorcluster, "instrument handle out"=w139:refnum<k15>)  [unwired: 6 in]
            n50 = property class="niDCPower"(reference=w139, error in=w155, "Active Channel"=w121, "Voltage Level Autorange"=w150, "Current Limit Autorange"=w150, "Source Delay"=w138, "Measure When"=w144) -> (reference out=w148:refnum<k15>, error out=w146:errorcluster)
            n51 = property class="niDCPower"(reference=w148, error in=w146, "Active Channel"=w121, "Transient Response"=w135, "Voltage GBW"=w143, "Voltage Compensation Freq"=w140, "Voltage Pole-Zero Ratio"=w132) -> (reference out=w147:refnum<k15>, error out=w145:errorcluster)
            n52 = call <instrlib>:"niDCPower Commit With Channels.vi"("error in (no error)"=w145, "channel name"=w121, "instrument handle"=w147) -> ("error out"=w161:errorcluster, "instrument handle out"=w160:refnum<k15>)  [unwired: 7 in]
            n53 = call <instrlib>:"niDCPower Initiate With Channels.vi"("error in (no error)"=w161, "channel name"=w121, "instrument handle"=w160) -> ("error out"=w134:errorcluster, "instrument handle out"=w142:refnum<k15>)  [unwired: 7 in]
            n54 = Bundle By Name(cluster=w116, "Source channel name"=w121, "Source out"=w142) -> (w141:T4)
          }
          frame "InitializeLoadConfiguration" {
            w196 = 1 items=["Off", "On"] ("Source:DC Current:Current Level Autorange")
            w205 = T8 1030 items=["Source Complete Event"=1030, "Measure Complete Event"=1031, "Sequence Iteration Complete Event"=1032, "Sequence Engine Done Event"=1033, "Pulse Complete Event"=1051, "Ready For Pulse Trigger Event"=1052] ("event")
            w208 = 1007 items=["DC Voltage"=1006, "DC Current"=1007, "Pulse Voltage"=1049, "Pulse Current"=1050] ("Source:Output Function")
            w209 = 1020 items=["Single Point"=1020, "Sequence"=1021] ("Source:Source Mode")
            # "1.Initalizing the Load configuration by setting the current level to current set point 1 with DUT setup time.\n2.This is to set the DUT to an inital state before sequencing\n3.Taking out trigger for setting different delays for different voltage level."
            n55 = Unbundle By Name(w178) -> ("dcpower session reservation"=w173:refnum<class "Session Reservation.lvclass">)
            n56 = Unbundle By Name(w195) -> ("Load pin name"=w174:string)
            n57 = call-poly <vilib>:"Get Connections.vi"("error in"=w176, "pin or relay name"=w174, "session reservation in"=w173) -> ("error out"=w175:errorcluster, "connection"=w172:T11)  [unwired: 6 in, 1 out]
            n58 = Unbundle By Name(w195) -> ("Load sense"=w179:i32, "Load current set point 1"=w186:dbl, "Load voltage limit range"=w187:dbl, "DUT setup time"=w194:dbl)
            n59 = Unbundle By Name(w172) -> ("session"=w171:refnum<k15>, "connection.channel"=w170:string)
            n60 = Unbundle By Name(w195) -> ("Load transient response"=w183:i32, "Load current gain bandwidth"=w193:dbl, "Load current compensation frequency"=w192:dbl, "Load current pole-zero ratio"=w191:dbl)
            n61 = call <instrlib>:"niDCPower Configure Sense.vi"("error in (no error)"=w175, "sense"=w179, "channel name"=w170, "instrument handle"=w171) -> ("error out"=w201:errorcluster, "instrument handle out"=w202:refnum<k15>)  [unwired: 6 in]
            n62 = property class="niDCPower"(reference=w202, error in=w201, "Active Channel"=w170, "Source Mode"=w209, "Output Function"=w208, "Current Level"=w186, "Voltage Limit Range"=w187, "Current Level Autorange"=w196, "Source Delay"=w194) -> (reference out=w198:refnum<k15>, error out=w197:errorcluster)
            n63 = property class="niDCPower"(reference=w198, error in=w197, "Active Channel"=w170, "Transient Response"=w183, "Current GBW"=w193, "Current Compensation Freq"=w192, "Current Pole-Zero Ratio"=w191) -> (reference out=w185:refnum<k15>, error out=w184:errorcluster)
            n64 = call <instrlib>:"niDCPower Commit With Channels.vi"("error in (no error)"=w184, "channel name"=w170, "instrument handle"=w185) -> ("error out"=w199:errorcluster, "instrument handle out"=w200:refnum<k15>)  [unwired: 7 in]
            n65 = call <instrlib>:"niDCPower Initiate With Channels.vi"("error in (no error)"=w199, "channel name"=w170, "instrument handle"=w200) -> ("error out"=w207:errorcluster, "instrument handle out"=w206:refnum<k15>)  [unwired: 7 in]
            n66 = call <instrlib>:"niDCPower Wait For Event With Channels.vi"("error in (no error)"=w207, "event"=w205, "channel name"=w170, "instrument handle"=w206) -> ("error out"=w204:errorcluster, "instrument handle out"=w203:refnum<k15>)  [unwired: 6 in]
            n67 = call <instrlib>:"niDCPower Abort With Channels.vi"("error in (no error)"=w204, "channel name"=w170, "instrument handle"=w203) -> ("error out"=w182:errorcluster, "instrument handle out"=w190:refnum<k15>)  [unwired: 7 in]
            n68 = Match Pattern(string=w170, regular expression="/") -> (before substring=w167:string, after substring=w166:string)  [unwired: 1 in, 2 out]
            n69 = call "Build Trigger Terminal.vi"("error in (no error)"=w182, "Trigger/Event Name"="StartTrigger" ("Trigger Type"), "Channel Name"=w166, "Resource Name"=w167) -> ("error out"=w169:errorcluster, "Terminal Name"=w181:string)  [unwired: 6 in]
            n70 = call "Build Trigger Terminal.vi"("error in (no error)"=w169, "Trigger/Event Name"="SourceCompleteEvent" ("Trigger Type"), "Channel Name"=w166, "Resource Name"=w167) -> ("error out"=w168:errorcluster, "Terminal Name"=w164:string)  [unwired: 6 in]
            n71 = Bundle By Name(cluster=w178, "Load channel name"=w170, "Load out"=w190, "Measure terminal name"=w181, "Scope ref trigger source"=w164) -> (w189:T4)
          }
          frame "ConfigureAndInitiateScope" {
            w210 = 2  # Number of records
            w230 = TRUE  # Enable TClk
            # "Perform scope measurements twice around the rising and falling edges of the load current."
            n72 = Unbundle By Name(w216) -> ("Pin Names for Scope"=w212:string[], "vertical range"=w229:dbl[], "vertical offset"=w228:dbl[], "probe attenuation"=w227:dbl[], "vertical coupling"=w226:T3[], "channel enabled"=w225:bool[], "input impedance"=w224:u32[], "max input frequency"=w223:dbl[], "min sample rate"=w222:dbl[], "reference position"=w221:dbl[], "min record length"=w220:i32[], "enforce realtime"=w219:bool[])
            n73 = Unbundle By Name(w211) -> ("Scope ref trigger source"=w213:string)
            n74 = Bundle By Name(cluster=w211, "Number of records"=w210, "Enable TClk"=w230) -> (w215:T4)
            n75 = Array Size(array=w219) -> (size(s)=w218:i32)
            n76 = Initialize Array(w210, w218) -> (w217:i32[])
            n77 = Build Cluster Array(w229, w228, w227, w226, w225, w224, w223, w222, w221, w220, w217, w219) -> (w214:T14)
            n78 = case shown="False" w230 {
              tunnel: w235 -> [w239 w279]
              tunnel: w215 -> [w249 w286]
              tunnel: [w248 w280] -> w233
              tunnel: [w247 w287] -> w234
              tunnel: w232 -> [w240 w278]
              tunnel: [w240 w278] -> w231
              tunnel: w214 -> [w236 w276]
              tunnel: w213 -> [w238 w275]
              tunnel: w212 -> [w237 w277]
              frame False {
                # "TClk has not been supported by grpc-device and cannot be used with the Measurement Plug-In APIs as of 2024 Q4.\nFor strict synchronization with TClk, you need to use the niScope Initialize with Options VI to initialize sessions."
                n79 = Array Size(array=w237) -> (size(s)=w241:i32)
                n80 = case shown="1.." w241 {
                  tunnel: w240 -> [_ w262]
                  tunnel: w239 -> [w250 w261]
                  tunnel: w237 -> [_ w255]
                  tunnel: [_ w254] -> w246
                  tunnel: [_ w253] -> w244
                  tunnel: [w250 w252] -> w243
                  tunnel: [_ w251] -> w242
                  frame 0, Default {
                  }
                  frame 1.. {
                    n81 = call-poly <vilib>:"Reserve Sessions.vi"("error in"=w261, "pin or relay names"=w255, "measurement context in"=w262) -> ("error out"=w260:errorcluster, "session reservation out"=w259:refnum<class "Session Reservation.lvclass">)  [unwired: 6 in, 1 out]
                    n82 = call-poly <vilib>:"Initialize Sessions.vi"("error in"=w260, "reset"=FALSE, "session reservation in"=w259) -> ("error out"=w258:errorcluster, "sessions"=w253:refnum<k15>[], "session reservation out"=w257:refnum<class "Session Reservation.lvclass">)  [unwired: 5 in, 1 out]
                    n83 = call-poly <vilib>:"Get Connections.vi"("error in"=w258, "pin or relay names"=w255, "session reservation in"=w257) -> ("error out"=w252:errorcluster, "connections"=w251:T15[], "session reservation out"=w254:refnum<class "Session Reservation.lvclass">)  [unwired: 6 in]
                  }
                }
                n84 = Bundle By Name(cluster=w249, "scope session reservation"=w246) -> (w248:T4)
                n85 = for {
                  tunnel: w242 -> [w274] mode=indexing
                  shift-right: [w267] -> w245
                  shift-left: w243 -> [w271]
                  tunnel: w238 -> [w268]
                  tunnel: w236 -> [w266] mode=indexing
                  n86 = Unbundle By Name(w274) -> ("session"=w273:refnum<k15>, "connection.channel"=w272:string)
                  n87 = call "Setup Scope.vi"("instrument handle"=w273, "channels"=w272, "Scope Parameters"=w266, "error in"=w271) -> ("instrument handle out"=w269:refnum<k15>, "error out"=w270:errorcluster)  [unwired: 10 in]
                  n88 = call-poly <instrlib>:"niScope Configure Trigger (poly).vi"("instrument handle"=w269, "trigger source"=w268, "error in"=w270) -> ("error out"=w267:errorcluster)  [unwired: 11 in, 1 out]
                }
                n89 = for {
                  tunnel: w244 -> [w263] mode=indexing
                  shift-right: [w264] -> w247
                  shift-left: w245 -> [w265]
                  n90 = call <instrlib>:"niScope Initiate Acquisition.vi"("instrument handle"=w263, "error in"=w265) -> ("error out"=w264:errorcluster)  [unwired: 12 in, 1 out]
                }
              }
              frame True {
                n91 = call-dynamic "Get Pin Map Context.vi"("error in"=w279, "measure call context in"=w278) -> ("error out"=w290:errorcluster, "pin map context"=w291:T16)  [unwired: 7 in, 1 out]
                n92 = Unbundle By Name(w291) -> ("pin map id"=w289:string)
                n93 = Build Path(name or relative path=w289) -> (appended path=w288:path)  [unwired: 1 in]
                n94 = call "Create Connection Map From Pin Map File.vi"("error in (no error)"=w290, "pin map file path"=w288) -> ("error out"=w283:errorcluster, "connection map"=w285:map{string, T5[]})  [unwired: 8 in]
                n95 = call "Create Scope Info Map for Each Site.vi"("error in (no error)"=w283, "parameters array"=w276, "Pin Names for Scope"=w277, "connection map"=w285) -> ("error out"=w282:errorcluster, "scope info map for each site"=w284:T17)  [unwired: 6 in]
                n96 = for {
                  tunnel: w275 -> [w295]
                  shift-right: [w294] -> w287
                  shift-left: w282 -> [w296]
                  tunnel: [w293] -> w281 mode=indexing
                  tunnel: w284 -> [w292] mode=indexing
                  # "Loop for multiple sites"
                  n97 = call "Initialize Configure Initiate Scope with TClk.vi"("error in (no error)"=w296, "ref trigger source"=w295, "scope info map"=w292) -> ("error out"=w294:errorcluster, "scope handles"=w293:refnum<k15>[])  [unwired: 7 in]
                }
                n98 = Bundle By Name(cluster=w286, "connection map"=w285, "instrument info map array"=w284, "Scope handles"=w281) -> (w280:T4)
              }
            }
          }
          frame "ConfigureLoadToSequence" {
            w301 = 1027 items=["Automatically after Source Complete"=1025, "On Demand"=1026, "On Measure Trigger"=1027] ("Measurement:Advanced:Measure When")
            w319 = 0 items=["Off", "On"] ("Source:DC Current:Current Level Autorange")
            w339 = T18 1028 items=["Seconds"=1028, "Powerline Cycles"=1029] ("aperture time units")
            w338 = T13 1007 items=["DC Voltage"=1006, "DC Current"=1007, "Pulse Voltage"=1049, "Pulse Current"=1050] ("output function")
            w340 = T8 1033 items=["Source Complete Event"=1030, "Measure Complete Event"=1031, "Sequence Iteration Complete Event"=1032, "Sequence Engine Done Event"=1033, "Pulse Complete Event"=1051, "Ready For Pulse Trigger Event"=1052] ("event")
            w341 = T9 1021 items=["Single Point"=1020, "Sequence"=1021] ("source mode")
            # "1.Initailizing load to sequence mode\n2.Defining the custom transient response for load current\n3.Defining the raising and falling slew rate for output current\n4.Configuring the load sequence to current set points"
            n99 = Unbundle By Name(w303) -> ("Load channel name"=w305:string, "Load out"=w334:refnum<k15>)
            n100 = Unbundle By Name(w311) -> ("Load current level range"=w318:dbl, "Load sample rate"=w353:dbl, "Load current delay t1"=w314:dbl, "Load current pulse duration"=w313:dbl, "Load current delay t2"=w312:dbl)
            n101 = call <instrlib>:"niDCPower Configure Source Mode With Channels.vi"("error in (no error)"=w330, "source mode"=w341, "channel name"=w305, "instrument handle"=w334) -> ("error out"=w345:errorcluster, "instrument handle out"=w344:refnum<k15>)  [unwired: 6 in]
            n102 = Compound Arithmetic op=ADD(w314, w313, w312) -> (w315:dbl)
            n103 = call <instrlib>:"niDCPower Configure Output Function.vi"("error in (no error)"=w345, "output function"=w338, "channel name"=w305, "instrument handle"=w344) -> ("error out"=w347:errorcluster, "instrument handle out"=w346:refnum<k15>)  [unwired: 6 in]
            n104 = Reciprocal(x=w353) -> (1/x=w348:dbl)
            n105 = Compound Arithmetic op=MULTIPLY(w353, w315) -> (w350:dbl)
            n106 = call <instrlib>:"niDCPower Configure Aperture Time.vi"("aperture time units"=w339, "error in (no error)"=w347, "aperture time"=w348, "channel name"=w305, "instrument handle"=w346) -> ("error out"=w336:errorcluster, "instrument handle out"=w335:refnum<k15>)  [unwired: 5 in]
            n107 = To Long Integer(number=w350) -> (32bit integer=w321:i32)
            n108 = Unbundle By Name(w311) -> ("Load transient response"=w320:i32, "Load current gain bandwidth"=w333:dbl, "Load current compensation frequency"=w332:dbl, "Load current pole-zero ratio"=w331:dbl, "Load current rising slew rate"=w317:dbl, "Load current falling slew rate"=w316:dbl, "Load current set point 1"=w328:dbl, "Load current set point 2"=w327:dbl, "Load current set point 1"=w326:dbl)
            n109 = property class="niDCPower"(reference=w335, error in=w336, "Active Channel"=w305, "Current Level Autorange"=w319, "Current Level Range"=w318, "Source Delay"=0.0 ("Source:Advanced:Source Delay"), "Measure Record Length"=w321) -> (reference out=w355:refnum<k15>, error out=w356:errorcluster)
            n110 = Unbundle By Name(w303) -> ("Measure terminal name"=w302:string)
            n111 = Unbundle By Name(w311) -> ("Load current delay t1"=w310:dbl, "Load current pulse duration"=w309:dbl, "Load current delay t2"=w308:dbl)
            n112 = property class="niDCPower"(reference=w355, error in=w356, "Active Channel"=w305, "Transient Response"=w320, "Current GBW"=w333, "Current Compensation Freq"=w332, "Current Pole-Zero Ratio"=w331, "Current Level Rising Slew Rate"=w317, "Current Level Falling Slew Rate"=w316) -> (reference out=w357:refnum<k15>, error out=w358:errorcluster)
            n113 = Build Array(w328, w327, w326) -> (w325:dbl[])
            n114 = Build Array(w310, w309, w308) -> (w307:dbl[])
            n115 = call <instrlib>:"niDCPower Set Sequence.vi"("source delays"=w307, "error in (no error)"=w358, "values"=w325, "channel name"=w305, "instrument handle"=w357) -> ("error out"=w304:errorcluster, "instrument handle out"=w306:refnum<k15>)  [unwired: 5 in]
            n116 = call-poly <instrlib>:"niDCPower Configure Trigger With Channels (Poly).vi"("error in (no error)"=w304, "input terminal"=w302, "channel name"=w305, "instrument handle"=w306) -> ("error out"=w298:errorcluster, "instrument handle out"=w300:refnum<k15>)  [unwired: 6 in]
            n117 = property class="niDCPower"(reference=w300, error in=w298, "Measure When"=w301) -> (reference out=w299:refnum<k15>, error out=w297:errorcluster)
            n118 = call <instrlib>:"niDCPower Commit With Channels.vi"("error in (no error)"=w297, "channel name"=w305, "instrument handle"=w299) -> ("error out"=w354:errorcluster, "instrument handle out"=w349:refnum<k15>)  [unwired: 7 in]
            n119 = property class="niDCPower"(reference=w349, error in=w354, "Active Channel"=w305) -> (reference out=w343:refnum<k15>, error out=w342:errorcluster, "Measure Record dt"=w322:dbl)
            n120 = call <instrlib>:"niDCPower Initiate With Channels.vi"("error in (no error)"=w342, "channel name"=w305, "instrument handle"=w343) -> ("error out"=w352:errorcluster, "instrument handle out"=w351:refnum<k15>)  [unwired: 7 in]
            n121 = Bundle By Name(cluster=w303, "Measurement Results.dt"=w322, "No of samples to fetch"=w321) -> (w329:T4)
            n122 = call <instrlib>:"niDCPower Wait For Event With Channels.vi"("error in (no error)"=w352, "event"=w340, "channel name"=w305, "instrument handle"=w351) -> ("error out"=w323:errorcluster)  [unwired: 6 in, 1 out]
          }
          frame "PerformMeasurement" {
            # "1.Fetches the voltages and currents of both the PPS and E-Load as per numbers of samples fetched"
            n123 = Unbundle By Name(w382) -> ("Number of records"=w359:i32, "Enable TClk"=w381:bool, "scope session reservation"=w380:refnum<class "Session Reservation.lvclass">, "Scope handles"=w376:refnum<k15>[][], "instrument info map array"=w375:T17)
            n124 = Unbundle By Name(w364) -> ("Pin Names for Scope"=w379:string[], "channel enabled"=w378:bool[], "min record length"=w360:i32[])
            n125 = for {
              N: w359 -> [_]
              tunnel: w381 -> [w410]
              tunnel: w380 -> [w409]
              tunnel: w379 -> [w408]
              tunnel: w378 -> [w407]
              tunnel: w360 -> [w406]
              tunnel: w376 -> [w404]
              tunnel: w375 -> [w403]
              tunnel: [w402] -> w374 mode=concatenating
              tunnel: [w401] -> w373 mode=concatenating
              tunnel: [w399] -> w363 mode=concatenating
              shift-right: [w400] -> w371
              shift-left: w377 -> [w405]
              i -> [w398]
              n126 = case shown="False" w410 {
                tunnel: w405 -> [w414 w439]
                tunnel: w406 -> [w411 _]
                tunnel: w398 -> [w412 w436]
                tunnel: [w424 w438] -> w400
                tunnel: [w423 w437] -> w399
                tunnel: w404 -> [_ w440]
                tunnel: w403 -> [_ w435]
                tunnel: [w421 w434] -> w401
                tunnel: [w422 w433] -> w402
                tunnel: w409 -> [w418 _]
                tunnel: w408 -> [w417 _]
                tunnel: w407 -> [w416 _]
                frame False {
                  n127 = for {
                    tunnel: w417 -> [w432] mode=indexing
                    tunnel: w416 -> [w431] mode=indexing
                    tunnel: [w432] -> w420 mode=indexing if=w431
                  }
                  n128 = Array Size(array=w420) -> (size(s)=w419:i32)
                  n129 = case shown="1.." w419 {
                    tunnel: w414 -> [w425 w430]
                    tunnel: [_ w429] -> w413
                    tunnel: w418 -> [_ w428]
                    tunnel: w420 -> [_ w427]
                    tunnel: [w425 w426] -> w415
                    frame 0, Default {
                      # "Do nothing if Pin Names are empty."
                    }
                    frame 1.. {
                      n130 = call-poly <vilib>:"Get Connections.vi"("error in"=w430, "pin or relay names"=w427, "session reservation in"=w428) -> ("error out"=w426:errorcluster, "connections"=w429:T15[])  [unwired: 6 in, 1 out]
                    }
                  }
                  n131 = call "Fetch Waveforms for One Record.vi"("error in (no error)"=w415, "min record length"=w411, "fetch record number"=w412, "connections"=w413) -> ("error out"=w424:errorcluster, "waveforms"=w423:waveform(dbl)[], "sites"=w421:i32[], "pins or relay names"=w422:string[])  [unwired: 4 in]
                }
                frame True {
                  n132 = for {
                    tunnel: w440 -> [w448] mode=indexing
                    shift-right: [w445] -> w438
                    shift-left: w439 -> [w447]
                    tunnel: [w446] -> w437 mode=concatenating
                    tunnel: w436 -> [w444]
                    tunnel: w435 -> [w443] mode=indexing
                    tunnel: [w442] -> w433 mode=concatenating
                    tunnel: [w441] -> w434 mode=concatenating
                    # "Loop for multiple sites"
                    n133 = call "Fetch Waveforms for One Record with Scope Info Map.vi"("error in (no error)"=w447, "fetch record number"=w444, "scope info map"=w443, "Scope handles"=w448) -> ("error out"=w445:errorcluster, "waverforms"=w446:waveform(dbl)[], "sites"=w441:i32[], "pins"=w442:string[])  [unwired: 4 in]
                  }
                }
              }
            }
            n134 = Unbundle By Name(w382) -> ("Load out"=w390:refnum<k15>, "Load channel name"=w389:string, "No of samples to fetch"=w388:i32)
            n135 = call <instrlib>:"niDCPower Fetch Multiple.vi"("instrument handle"=w390, "channel name"=w389, "count (1)"=w388, "timeout (1.0)"=10.0, "error in (no error)"=w377) -> ("voltage measurements"=w385:dbl[], "current measurements"=w387:dbl[], "error out"=w372:errorcluster)  [unwired: 5 in, 3 out]
            n136 = Array Max & Min(array=w385) -> (max value=w383:dbl, min value=w384:dbl)  [unwired: 2 out]
            n137 = call "Concatenate Waveform Array.vi"("waveform array"=w363) -> ("waveform t0 array"=w369:dbl[], "waveform dt array"=w368:dbl[], "waveform length array"=w367:i32[], "concatenated waveform Y"=w370:dbl[])  [unwired: 11 in]
            n138 = Bundle By Name(cluster=w382, "Measurement Results.Overshoot load voltage"=w383, "Measurement Results.Undershoot load voltage"=w384, "Measurement Results.Load voltages"=w385, "Measurement Results.Load currents"=w387, "Measurement Results.waveform pins"=w374, "Measurement Results.waveform sites"=w373, "Measurement Results.waveform t0 array"=w369, "Measurement Results.waveform dt array"=w368, "Measurement Results.waveform length array"=w367, "Measurement Results.concatenated waveform Y"=w370) -> (w362:T4)
            n139 = Unbundle By Name(w362) -> ("Measurement Results"=w361:T1)
            n140 = Merge Errors(w372, w371) -> (w366:errorcluster)
            n141 = disable-structure shown="Disabled" {
              disable-tunnel: w366 -> [w396 w397]
              disable-tunnel: [w395 w397] -> w365
              disable-tunnel: w364 -> [w394 _]
              disable-tunnel: w363 -> [w393 _]
              disable-tunnel: w361 -> [w392 _]
              frame Disabled {
                n142 = call "Save Results to TDMS.vi"("measurement configuration"=w394, "measurement results"=w392, "Scope waveforms"=w393, "error in (no error)"=w396) -> ("error out"=w395:errorcluster)  [unwired: 15 in]
              }
              frame Enabled {
              }
            }
          }
          frame "Exit", Default {
            # "1. Aborts the channels\n2. Close all the opened sessions\n3. Updates the status if measurement is performed"
            n143 = Release Queue(queue=w456, error in (no error)=w455) -> (error out=w454:errorcluster)  [unwired: 1 in, 2 out]
            n144 = case shown="Error .." w454 {
              selector: w454 -> [w471 w514]
              tunnel: w450 -> [w470 w515]
              tunnel: [w463 w513] -> w451
              tunnel: ["The measurement is performed successfully" ("message") _] -> w452
              tunnel: w449 -> [w459 w498]
              frame No Error {
                # "Abort, close sessions and updates the status indicator on the operation performed"
                n145 = Unbundle By Name(w470) -> ("Enable TClk"=w462:bool, "Scope handles"=w460:refnum<k15>[][], "scope session reservation"=w461:refnum<class "Session Reservation.lvclass">, "dcpower session reservation"=w465:refnum<class "Session Reservation.lvclass">, "Source out"=w473:refnum<k15>, "Source channel name"=w475:string, "Load out"=w472:refnum<k15>, "Load channel name"=w474:string)
                n146 = call <instrlib>:"niDCPower Abort With Channels.vi"("error in (no error)"=w471, "channel name"=w474, "instrument handle"=w472) -> ("error out"=w476:errorcluster)  [unwired: 7 in, 1 out]
                n147 = call <instrlib>:"niDCPower Abort With Channels.vi"("error in (no error)"=w476, "channel name"=w475, "instrument handle"=w473) -> ("error out"=w467:errorcluster)  [unwired: 7 in, 1 out]
                n148 = call <vilib>:"Close Sessions.vi"("error in"=w467, "session reservation in"=w465) -> ("error out"=w466:errorcluster, "session reservation out"=w468:refnum<class "Session Reservation.lvclass">)  [unwired: 8 in]
                n149 = call <vilib>:"Unreserve Sessions.vi"("error in"=w466, "session reservation in"=w468) -> ("error out"=w464:errorcluster)  [unwired: 9 in]
                n150 = case shown="False" w462 {
                  tunnel: w464 -> [w482 w490]
                  tunnel: [w481 w489] -> w463
                  tunnel: w461 -> [w480 _]
                  tunnel: w459 -> [w479 _]
                  tunnel: w460 -> [_ w491]
                  frame False {
                    n151 = Unbundle By Name(w479) -> ("Pin Names for Scope"=w478:string[])
                    n152 = Array Size(array=w478) -> (size(s)=w477:i32)
                    n153 = case shown="1.." w477 {
                      tunnel: w482 -> [w483 w487]
                      tunnel: [w483 w485] -> w481
                      tunnel: w480 -> [_ w484]
                      frame 0, Default {
                      }
                      frame 1.. {
                        n154 = call <vilib>:"Close Sessions.vi"("error in"=w487, "session reservation in"=w484) -> ("error out"=w486:errorcluster, "session reservation out"=w488:refnum<class "Session Reservation.lvclass">)  [unwired: 8 in]
                        n155 = call <vilib>:"Unreserve Sessions.vi"("error in"=w486, "session reservation in"=w488) -> ("error out"=w485:errorcluster)  [unwired: 9 in]
                      }
                    }
                  }
                  frame True {
                    n156 = for {
                      tunnel: w491 -> [w494] mode=indexing
                      shift-right: [w492] -> w489
                      shift-left: w490 -> [w493]
                      n157 = for {
                        tunnel: w494 -> [w495] mode=indexing
                        shift-right: [w496] -> w492
                        shift-left: w493 -> [w497]
                        n158 = call <instrlib>:"niScope Close.vi"("instrument handle"=w495, "error in"=w497) -> ("error out"=w496:errorcluster)  [unwired: 13 in]
                      }
                    }
                  }
                }
              }
              frame Error {
                # "Resets the device with default values whenever there is an error"
                n159 = Unbundle By Name(w515) -> ("Enable TClk"=w499:bool, "Scope handles"=w500:refnum<k15>[][], "scope session reservation"=w501:refnum<class "Session Reservation.lvclass">, "dcpower session reservation"=w504:refnum<class "Session Reservation.lvclass">, "Source out"=w510:refnum<k15>, "Source channel name"=w509:string, "Load out"=w512:refnum<k15>, "Load channel name"=w511:string)
                n160 = call <instrlib>:"niDCPower Abort With Channels.vi"("channel name"=w511, "instrument handle"=w512) -> ("error out"=w516:errorcluster, "instrument handle out"=w519:refnum<k15>)  [unwired: 8 in]
                n161 = call <instrlib>:"niDCPower Reset With Channels.vi"("error in (no error)"=w516, "channel name"=w511, "instrument handle"=w519) -> ("error out"=w508:errorcluster)  [unwired: 7 in, 1 out]
                n162 = call <instrlib>:"niDCPower Abort With Channels.vi"("error in (no error)"=w508, "channel name"=w509, "instrument handle"=w510) -> ("error out"=w518:errorcluster, "instrument handle out"=w517:refnum<k15>)  [unwired: 7 in]
                n163 = call <instrlib>:"niDCPower Reset With Channels.vi"("error in (no error)"=w518, "channel name"=w509, "instrument handle"=w517) -> ("error out"=w506:errorcluster)  [unwired: 7 in, 1 out]
                n164 = call <vilib>:"Close Sessions.vi"("error in"=w506, "session reservation in"=w504) -> ("error out"=w505:errorcluster, "session reservation out"=w507:refnum<class "Session Reservation.lvclass">)  [unwired: 8 in]
                n165 = call <vilib>:"Unreserve Sessions.vi"("error in"=w505, "session reservation in"=w507) -> ("error out"=w503:errorcluster)  [unwired: 9 in]
                n166 = case shown="False" w499 {
                  tunnel: w503 -> [w525 w533]
                  tunnel: [w524 w532] -> w502
                  tunnel: w501 -> [w523 _]
                  tunnel: w498 -> [w522 _]
                  tunnel: w500 -> [_ w534]
                  frame False {
                    n167 = Unbundle By Name(w522) -> ("Pin Names for Scope"=w521:string[])
                    n168 = Array Size(array=w521) -> (size(s)=w520:i32)
                    n169 = case shown="1.." w520 {
                      tunnel: w525 -> [w526 w530]
                      tunnel: [w526 w528] -> w524
                      tunnel: w523 -> [_ w527]
                      frame 0, Default {
                      }
                      frame 1.. {
                        n170 = call <vilib>:"Close Sessions.vi"("error in"=w530, "session reservation in"=w527) -> ("error out"=w529:errorcluster, "session reservation out"=w531:refnum<class "Session Reservation.lvclass">)  [unwired: 8 in]
                        n171 = call <vilib>:"Unreserve Sessions.vi"("error in"=w529, "session reservation in"=w531) -> ("error out"=w528:errorcluster)  [unwired: 9 in]
                      }
                    }
                  }
                  frame True {
                    n172 = for {
                      tunnel: w534 -> [w537] mode=indexing
                      shift-right: [w535] -> w532
                      shift-left: w533 -> [w536]
                      n173 = for {
                        tunnel: w537 -> [w538] mode=indexing
                        shift-right: [w539] -> w535
                        shift-left: w536 -> [w540]
                        n174 = call <instrlib>:"niScope Close.vi"("instrument handle"=w538, "error in"=w540) -> ("error out"=w539:errorcluster)  [unwired: 13 in]
                      }
                    }
                  }
                }
                n175 = Merge Errors(w514, w502) -> (w513:errorcluster)
              }
            }
            n176 = Bundle By Name(cluster=w450, "Measurement Results.Status"=w452) -> (w453:T4)
          }
        }
      }
    }
    frame "Power off the DUT" {
      # "Stops generation on the output channel and resets the channels to default values"
      n177 = Unbundle By Name(w581) -> ("Source pin name"=w563:string, "Load pin name"=w565:string)
      n178 = Build Array(w563, w565) -> (w571:string[])
      n179 = call-poly <vilib>:"Reserve Sessions.vi"("timeout (ms)"=60000, "error in"=w572, "pin or relay names"=w571, "measurement context in"=w570) -> ("error out"=w577:errorcluster, "session reservation out"=w576:refnum<class "Session Reservation.lvclass">)  [unwired: 5 in, 1 out]
      n180 = call-poly <vilib>:"Initialize Sessions.vi"("error in"=w577, "session reservation in"=w576) -> ("error out"=w575:errorcluster, "session reservation out"=w574:refnum<class "Session Reservation.lvclass">)  [unwired: 6 in, 2 out]
      n181 = call-poly <vilib>:"Get Connections.vi"("error in"=w575, "pin or relay name"=w565, "session reservation in"=w574) -> ("error out"=w568:errorcluster, "connection"=w569:T11, "session reservation out"=w562:refnum<class "Session Reservation.lvclass">)  [unwired: 6 in]
      n182 = Unbundle By Name(w569) -> ("session"=w566:refnum<k15>, "connection.channel"=w567:string)
      n183 = call <instrlib>:"niDCPower Configure Output Enabled.vi"("error in (no error)"=w568, "output enabled"=FALSE, "channel name"=w567, "instrument handle"=w566) -> ("error out"=w583:errorcluster, "instrument handle out"=w584:refnum<k15>)  [unwired: 6 in]
      n184 = call <instrlib>:"niDCPower Reset With Channels.vi"("error in (no error)"=w583, "channel name"=w567, "instrument handle"=w584) -> ("error out"=w564:errorcluster)  [unwired: 7 in, 1 out]
      n185 = call-poly <vilib>:"Get Connections.vi"("error in"=w564, "pin or relay name"=w563, "session reservation in"=w562) -> ("error out"=w551:errorcluster, "connection"=w561:T11, "session reservation out"=w557:refnum<class "Session Reservation.lvclass">)  [unwired: 6 in]
      n186 = Unbundle By Name(w561) -> ("session"=w554:refnum<k15>, "connection.channel"=w550:string)
      n187 = call <instrlib>:"niDCPower Configure Output Enabled.vi"("error in (no error)"=w551, "output enabled"=FALSE, "channel name"=w550, "instrument handle"=w554) -> ("error out"=w552:errorcluster, "instrument handle out"=w553:refnum<k15>)  [unwired: 6 in]
      n188 = call <instrlib>:"niDCPower Reset With Channels.vi"("error in (no error)"=w552, "channel name"=w550, "instrument handle"=w553) -> ("error out"=w556:errorcluster)  [unwired: 7 in, 1 out]
      n189 = call <vilib>:"Close Sessions.vi"("error in"=w556, "session reservation in"=w557) -> ("error out"=w559:errorcluster, "session reservation out"=w560:refnum<class "Session Reservation.lvclass">)  [unwired: 8 in]
      n190 = call <vilib>:"Unreserve Sessions.vi"("error in"=w559, "session reservation in"=w560) -> ("error out"=w558:errorcluster)  [unwired: 9 in]
      n191 = Bundle By Name(cluster=w580, "Measurement Results.Status"="The DUT is powered OFF" ("message")) -> (w578:T4)
    }
  }
  "error out" <- w1
  "measure call context out" <- w2
  n192 = Unbundle By Name(w10) -> ("Measurement Results"=→"measurement results":T1)
